vi "dsdll_get_exe_path.vi"() -> (0 "top level VI or exe":path, 1 "directory path":path, 2 "application root path":path, 3 "full path":path)   [LabVIEW 2018, in "dsdll.lvlib"]
doc: "Retrieves various paths related to the application."
uses:
  dsdll.lvlib
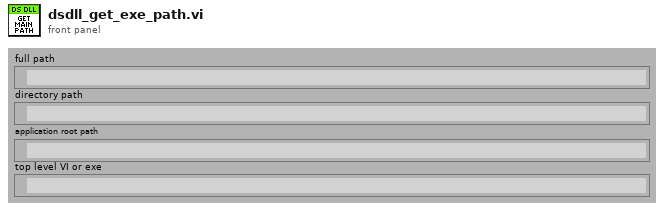
[diagram p1: front panel]
types:
  T1 = enum32{"invalid app kind", "Development System", "Run Time System", "Student Edition", "Embedded LabVIEW", "Evaluation", "Custom"}
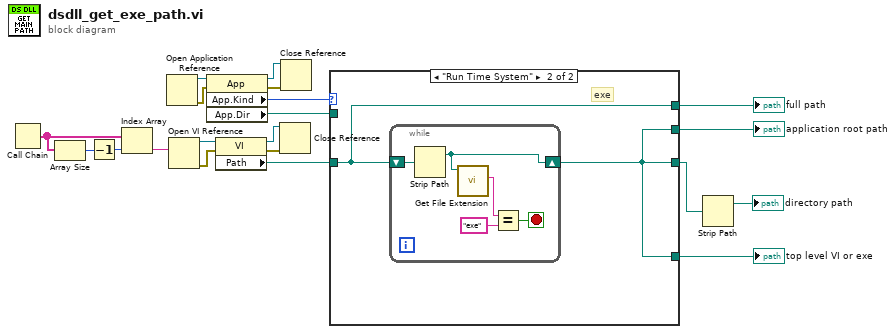
[diagram p0: block diagram]
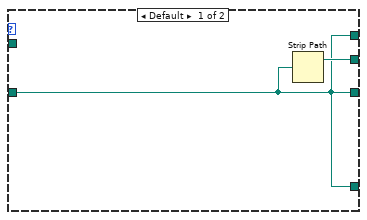
[diagram p2: hidden frame]
diagram:
  n1 = Call Chain() -> (call chain=w13:string[])
  n2 = Array Size(array=w13) -> (size(s)=w14:i32)
  n3 = Decrement(x=w14) -> (x-1=w12:i32)
  n4 = Index Array(array=w13, index=w12) -> (element=w11:string)
  n5 = Open Application Reference() -> (0:w5:errorcluster, 3:w18:refnum<vi>)  [unwired: 4 in]
  n6 = Open VI Reference(vi path=w11) -> (vi reference=w19:refnum<vi>, error out=w20:errorcluster)  [unwired: 5 in]
  n7 = property class="App"(reference=w18, error in=w5) -> (reference out=w8:refnum<vi>, error out=w9:errorcluster, "App.Kind"=w17:T1, "App.Dir"=w3:path)
  n8 = property class="VI"(reference=w19, error in=w20) -> (reference out=w6:refnum<vi>, error out=w7:errorcluster, "Path"=w16:path)
  n9 = Close Reference(reference=w6, error in (no error)=w7) -> ()  [unwired: 1 out]
  n10 = Close Reference(reference=w8, error in (no error)=w9) -> ()  [unwired: 1 out]
  n11 = case shown="\"Run Time System\"" w17 {
    tunnel: w16 -> [w21 w24]
    tunnel: [w21 w23] -> w15
    tunnel: [w22 w23] -> w4
    tunnel: w3 -> [_ _]
    tunnel: [w21 w24] -> w2
    tunnel: [w21 w23] -> w1
    frame Default {
      n12 = Strip Path(path=w21) -> (stripped path=w22:path)  [unwired: 1 out]
    }
    frame "Run Time System" {
      # "exe"
      n13 = while {
        shift-right: [w25] -> w23
        shift-left: w24 -> [w26]
        stop <- w27 stop-if-true
        n14 = Strip Path(path=w26) -> (stripped path=w25:path)  [unwired: 1 out]
        n15 = call <vilib>:"Get File Extension.vi"("file"=w25) -> ("lowercase file extension"=w29:string)  [unwired: 6 in, 4 out]
        n16 = Equal?(x=w29, y="exe") -> (x = y?=w27:bool)
      }
    }
  }
  "full path" <- w2
  "application root path" <- w4
  "top level VI or exe" <- w1
  n17 = Strip Path(path=w15) -> (stripped path=→"directory path":path)  [unwired: 1 out]
